vi "Draw Cursor.vi"(4 "Parse State":T1, 6 "Color":u32(colorbox), 8 "Font":T7, 11 "Picture In":picture) -> (3 "Picture":picture)   [LabVIEW 2020, in "Terminal.lvlib" / "Terminal.lvclass"]
uses:
  Terminal.lvclass
  Parse State.ctl
  Buffer State.ctl
  Cursor.ctl
  Position.ctl
  Text Attributes.ctl
  Buffer.ctl
  Terminal.lvclass/Terminal.ctl
  Terminal.lvlib
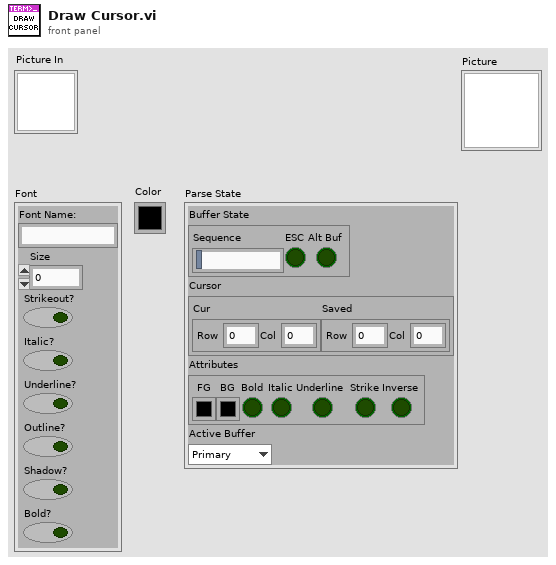
[diagram p1: front panel]
types:
  T1 = typedef "Terminal.lvlib/Terminal.lvclass/Parse State.ctl" = cluster{"Buffer State":T2, "Cursor":T3, "Attributes":T5, "Active Buffer":T6}
  T2 = typedef "Terminal.lvlib/Terminal.lvclass/Buffer State.ctl" = cluster{"Sequence":string, "ESC":bool, "Alt Buf":bool}
  T3 = typedef "Terminal.lvlib/Terminal.lvclass/Cursor.ctl" = cluster{"Cur":T4, "Saved":T4}
  T4 = typedef "Terminal.lvlib/Terminal.lvclass/Position.ctl" = cluster{"Row":i32, "Col":i32}
  T5 = typedef "Terminal.lvlib/Text Attributes.ctl" = cluster{"FG":u32, "BG":u32, "Bold":bool, "Italic":bool, "Underline":bool, "Strike":bool, "Inverse":bool}
  T6 = typedef "Terminal.lvlib/Buffer.ctl" = enum16{"Primary", "Alternate"}
  T7 = cluster{"Font Name:":string, "Size":i16, "Strikeout?":bool, "Italic?":bool, "Underline?":bool, "Outline?":bool, "Shadow?":bool, "Bold?":bool}
  T8 = cluster{"left":i16, "top":i16, "right":i16, "bottom":i16}
  T9 = enum16{"User-specified Font", "Application Font", "System Font", "Dialog Font"}
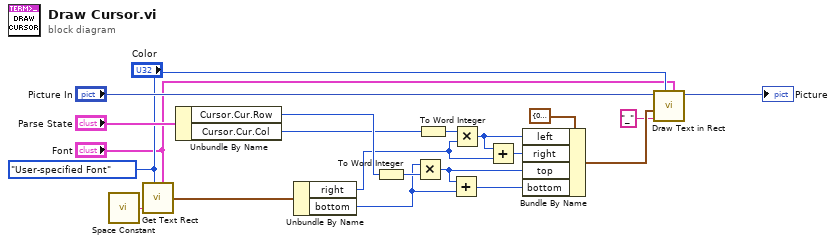
[diagram p0: block diagram]
diagram:
  w4 = T9."User-specified Font" ("desired font(Application)")
  n1 = call <vilib>:"Space Constant.vi"() -> ("String"=w19:string)
  n2 = call <vilib>:"Get Text Rect.vi"("desired font(Application)"=w4, "text"=w19, "[user-specified font]"="Font") -> ("rect"=w20:T8)  [unwired: 6 in]
  n3 = Unbundle By Name("Parse State") -> ("Cursor.Cur.Row"=w16:i32, "Cursor.Cur.Col"=w10:i32)
  n4 = Unbundle By Name(w20) -> ("right"=w7:i16, "bottom"=w15:i16)
  n5 = To Word Integer(number=w16) -> (16bit integer=w17:i16)
  n6 = Multiply(x=w15, y=w17) -> (x*y=w9:i16)
  n7 = To Word Integer(number=w10) -> (16bit integer=w13:i16)
  n8 = Add(x=w9, y=w15) -> (x+y=w8:i16)
  n9 = Multiply(x=w13, y=w7) -> (x*y=w11:i16)
  n10 = Add(x=w11, y=w7) -> (x+y=w12:i16)
  n11 = Bundle By Name(cluster=T8 {"left"=0, "top"=0, "right"=0, "bottom"=0} ("rect"), "left"=w11, "right"=w12, "top"=w9, "bottom"=w8) -> (w2:T8)
  n12 = call <vilib>:"Draw Text in Rect.vi"("[user-specified font]"="Font", "desired font(Application)"=w4, "text"="_", "rect"=w2, "picture"="Picture In") -> ("new picture"=→"Picture":picture)  [unwired: 6 in]
